vi "_Highlight CSM Scripts(StringConstant).vi"(8 "error in (no error)":errorcluster, 11 "Reference Out":refnum<vi>) -> (0 "error out":errorcluster)   [LabVIEW 2017]
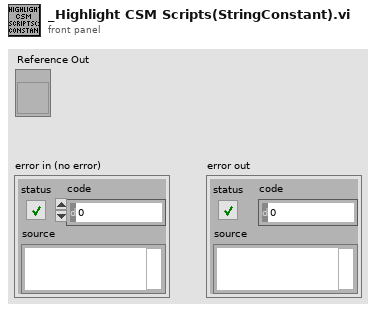
[diagram p1: front panel]
types:
  T1 = cluster{"Text.Selection:Start":u32, "Text.Selection:End":u32, "cb":u32, "underline":bool, "Italic":bool, "Bold":bool}[]
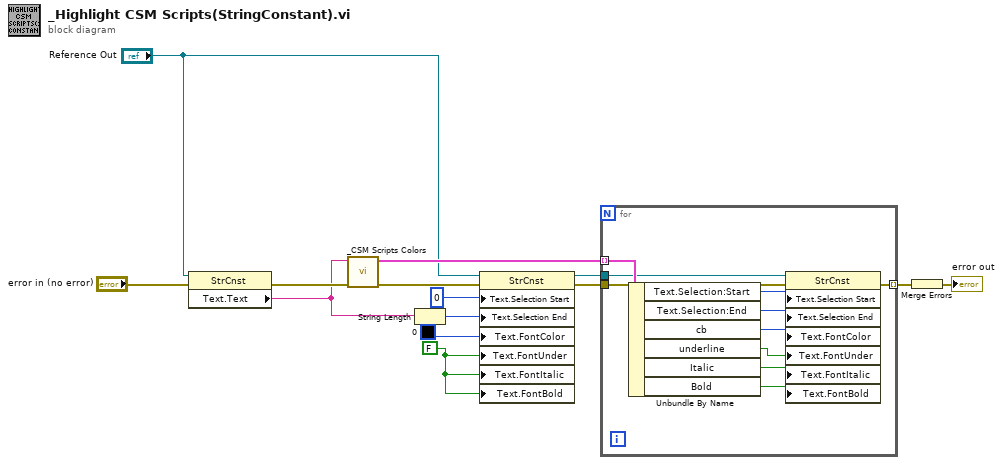
[diagram p0: block diagram]
diagram:
  w2 = FALSE ("Text.Font:Underline")
  n1 = property class="StrCnst"(reference="Reference Out", error in="error in (no error)") -> (error out=w12:errorcluster, "Text.Text"=w10:string)  [unwired: 1 out]
  n2 = call "_CSM Scripts Colors.vi"("Error In"=w12, "Value"=w10) -> ("error out"=w6:errorcluster, "Array"=w13:T1)  [unwired: 8 in]
  n3 = String Length(string=w10) -> (length=w4:i32)
  n4 = property class="StrCnst"(reference="Reference Out", error in=w6, "Text.Selection Start"=u32 0 ("Text.Selection:Start"), "Text.Selection End"=w4, "Text.FontColor"=u32 0, "Text.FontUnder"=w2, "Text.FontItalic"=w2, "Text.FontBold"=w2) -> (reference out=w8:refnum<vi>, error out=w9:errorcluster)
  n5 = for {
    tunnel: w8 -> [w23]
    tunnel: w9 -> [w19]
    tunnel: w13 -> [w24] mode=indexing
    tunnel: [w18] -> w11 mode=indexing
    n6 = Unbundle By Name(w24) -> ("Text.Selection:Start"=w22:u32, "Text.Selection:End"=w21:u32, "cb"=w20:u32, "underline"=w17:bool, "Italic"=w16:bool, "Bold"=w15:bool)
    n7 = property class="StrCnst"(reference=w23, error in=w19, "Text.Selection Start"=w22, "Text.Selection End"=w21, "Text.FontColor"=w20, "Text.FontUnder"=w17, "Text.FontItalic"=w16, "Text.FontBold"=w15) -> (error out=w18:errorcluster)  [unwired: 1 out]
  }
  n8 = Merge Errors(w11) -> (→"error out":errorcluster)
